vi "Item Ref to BaseNodeType.vi"(8 "error in (no error)":errorcluster, 11 "item ref in":T1 format="%.0x") -> (0 "error out":errorcluster, 2 "BaseNodeType":refnum<k24>, 3 "item ref out":T1 format="%.0x")   [LabVIEW 2017, in "Import Export.lvlib"]
uses:
  Import Export.lvlib
  <vilib>/NI Veristand/Custom Device API/Custom Device Item Ref.ctl
  NationalInstruments.VeriStand.SystemStorage
  NationalInstruments.VeriStand.SystemDefinitionAPI
  <vilib>/NI VeriStand/Custom Device API/Custom Device API.lvlib
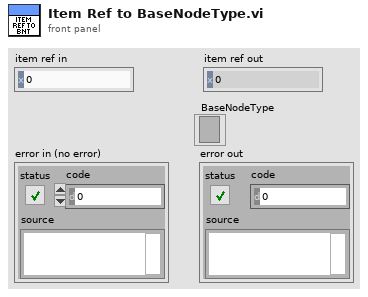
[diagram p1: front panel]
types:
  T1 = typedef "Custom Device API.lvlib/Custom Device Item Ref.ctl" = u64
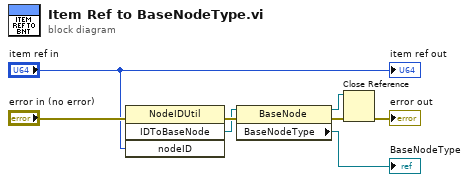
[diagram p0: block diagram]
diagram:
  n1 = invoke class="NodeIDUtil" method="IDToBaseNode"(error in="error in (no error)", "nodeID"="item ref in") -> (error out=w8:errorcluster, "IDToBaseNode"=w7:refnum<k24>)  [unwired: 2 in, 2 out]
  n2 = property class="BaseNode"(reference=w7, error in=w8) -> (reference out=w5:refnum<k24>, error out=w3:errorcluster, "BaseNodeType"=→"BaseNodeType":refnum<k24>)
  n3 = Close Reference(reference=w5, error in (no error)=w3) -> (error out=→"error out":errorcluster)
  "item ref out" <- "item ref in"
